vi "单轴控制.vi"() -> ()   [LabVIEW 2011]
panel:
  in  "方向":u16
  in  "停止":bool
  in  "运行":bool
  in  "速度":dbl
  in  "使能":bool
  in  "退出":bool
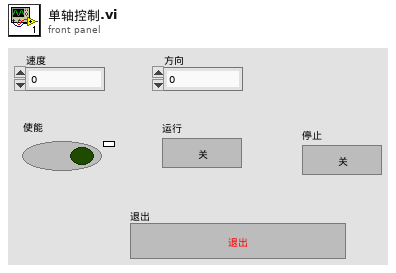
[diagram p1: front panel]
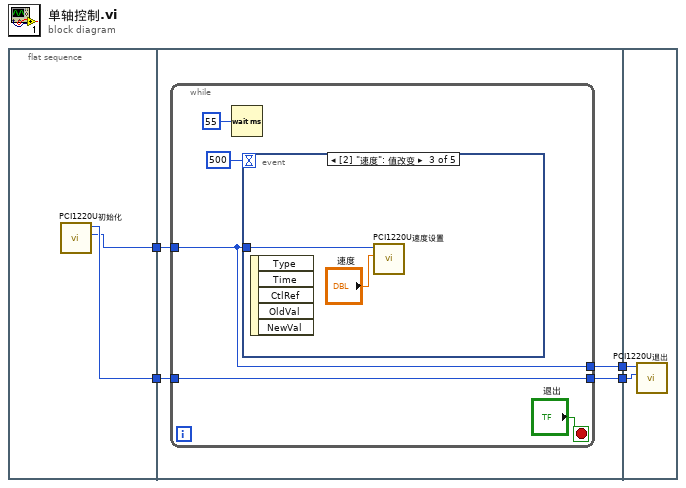
[diagram p0: block diagram]
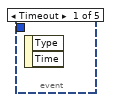
[diagram p2: hidden frame]
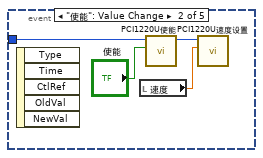
[diagram p3: hidden frame]
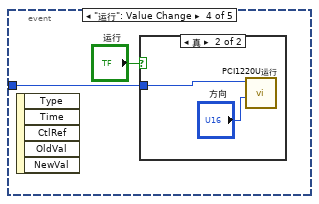
[diagram p4: hidden frame]
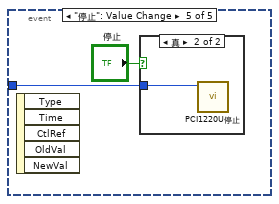
[diagram p6: hidden frame]
diagram:
  n1 = flat-sequence {
    tunnel: [w6] -> w2
    tunnel: [w5] -> w1
    tunnel: [w10] -> w4
    tunnel: [w9] -> w3
    tunnel: w2 -> [w8]
    tunnel: w1 -> [w7]
    tunnel: w4 -> [w30]
    tunnel: w3 -> [w29]
    frame #0 {
      n2 = call "PCI1220U初始化.vi"() -> ("AxisHandle OUT"=w5:u32, "DeviceHandle"=w6:u32)  [unwired: 8 in, 2 out]
    }
    frame #1 {
      n3 = while {
        tunnel: w8 -> [w13]
        tunnel: [w13] -> w9
        tunnel: w7 -> [w12]
        tunnel: [w12] -> w10
        stop <- "退出" stop-if-true
        n4 = Wait (ms)(milliseconds to wait=u32 55 ("等待时间（毫秒）")) -> ()  [unwired: 1 out]
        n5 = event shown="[2] \"速度\": 值改变" {
          selector: _ -> [_ _ _ _ _]
          dyn-events: _ -> [_ _ _ _ _]
          timeout: 500 -> [_ _ _ _ _]
          tunnel: w12 -> [_ w19 w21 w23 w26]
          event Timeout {
            n6 = event-data() -> ()  [unwired: 1 in, 2 out]
          }
          event "使能": Value Change {
            n7 = event-data() -> ()  [unwired: 1 in, 5 out]
            n8 = local read "速度"() -> (w16:dbl)
            n9 = call "PCI1220U使能.vi"("使能"="使能", "AxisHandle IN"=w19) -> ("AxisHandle OUT"=w17:u32)  [unwired: 9 in]
            n10 = call "PCI1220U速度设置.vi"("Change Velocity"=w16, "AxisHandle IN"=w17) -> ()  [unwired: 9 in, 1 out]
          }
          event "速度": Value Change {
            n11 = event-data() -> ()  [unwired: 1 in, 5 out]
            n12 = call "PCI1220U速度设置.vi"("Change Velocity"="速度", "AxisHandle IN"=w21) -> ()  [unwired: 9 in, 1 out]
          }
          event "运行": Value Change {
            n13 = event-data() -> ()  [unwired: 1 in, 5 out]
            n14 = case shown="真" "运行" {
              tunnel: w23 -> [_ w25]
              frame False {
              }
              frame True {
                n15 = call "PCI1220U运行.vi"("方向"="方向", "AxisHandle IN"=w25) -> ()  [unwired: 9 in, 1 out]
              }
            }
          }
          event "停止": Value Change {
            n16 = event-data() -> ()  [unwired: 1 in, 5 out]
            n17 = case shown="真" "停止" {
              tunnel: w26 -> [_ w28]
              frame False {
              }
              frame True {
                n18 = call "PCI1220U停止.vi"("AxisHandle IN"=w28) -> ()  [unwired: 9 in, 2 out]
              }
            }
          }
        }
      }
    }
    frame #2 {
      n19 = call "PCI1220U退出.vi"("DeviceHandle IN"=w29, "AxisHandle IN"=w30) -> ()  [unwired: 10 in]
    }
  }
